vi "Binary to ASCII hash.vi"(1 "Binary hash string":string) -> (0 "ASCII hash string":string)   [LabVIEW 2009]
doc: "This VI converts a binary hash as returned by OpenG hash functions to a human readable ASCII hash"
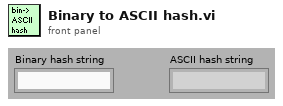
[diagram p1: front panel]
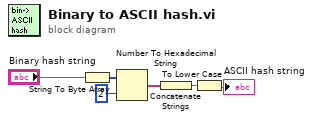
[diagram p0: block diagram]
diagram:
  n1 = String To Byte Array(string="Binary hash string") -> (unsigned byte array=w1:u8[])
  n2 = Number To Hexadecimal String(1:i16 2 ("width (-)"), 2:w1) -> (0:w2:string[])
  n3 = Concatenate Strings(w2) -> (w3:string)
  n4 = To Lower Case(string=w3) -> (all lower case string=→"ASCII hash string":string)
